vi "ReadVIInternal.vi"(1 "vi path":path) -> (0 "output cluster":T13)   [LabVIEW 2014]
uses:
  <vilib>/Utility/miscctls.llb/LVBoundsTypeDef.ctl
  <vilib>/Utility/miscctls.llb/LVPositionTypeDef.ctl
  <vilib>/Utility/miscctls.llb/LVRectTypeDef.ctl
  <vilib>/Utility/miscctls.llb/LVBreakpointStatusEnum.ctl
  <vilib>/Utility/miscctls.llb/LVDataSocketStatusTypeDef.ctl
  <vilib>/Utility/miscctls.llb/LVKeyNavTypeDef.ctl
  <vilib>/Utility/miscctls.llb/LVMinMaxIncTypeDef.ctl
  <vilib>/Utility/miscctls.llb/LVKeyTypeDef.ctl
  <vilib>/numeric/LVNumericRepresentation.ctl
  <vilib>/Utility/miscctls.llb/LVOutOfRangeActionTypeDef.ctl
  <vilib>/Utility/miscctls.llb/LVStringsAndValuesArrayTypeDef.ctl
  <vilib>/Utility/miscctls.llb/LVParallelSchedulesEnum.ctl
  <vilib>/Utility/traverseref.llb/VI Scripting - Traverse.lvlib
types:
  T1 = typedef "LVBoundsTypeDef.ctl" = cluster{"Width":u32, "Height":u32}
  T2 = typedef "LVPositionTypeDef.ctl" = cluster{"Left":i32, "Top":i32}
  T3 = typedef "LVRectTypeDef.ctl" = cluster{"Left":i16, "Top":i16, "Right":i16, "Bottom":i16}
  T4 = typedef "LVBreakpointStatusEnum.ctl" = enum8{"Cleared Break", "Enabled Break", "Disabled Break"}
  T5 = typedef "LVDataSocketStatusTypeDef.ctl" = cluster{"Code":enum32{"Invalid Status", "Unconnected", "Active", "Idle", "Error", "Connecting"}, "Text":string}
  T6 = typedef "LVKeyNavTypeDef.ctl" = cluster{"Control":bool, "Shift":bool, "Key":string}
  T7 = typedef "LVMinMaxIncTypeDef.ctl" = cluster{"Minimum":dbl, "Maximum":dbl, "Increment":dbl}
  T8 = typedef "LVKeyTypeDef.ctl" = cluster{"Focus":bool, "Control":bool, "Shift":bool, "Key":string}
  T9 = typedef "LVNumericRepresentation.ctl" = enum32{"Extended Precision", "Double Precision", "Single Precision", "Long", "Word", "Byte", "Unsigned Long", "Unsigned Word", "Unsigned Byte", "Complex Extended", "Complex Double", "Complex Single", "Quad", "Unsigned Quad", "Fixed-Point"}
  T10 = typedef "LVOutOfRangeActionTypeDef.ctl" = cluster{"Out of Range Action Minimum":u8, "Out of Range Action Maximum":u8, "Out of Range Action Increment":u8}
  T11 = typedef "LVStringsAndValuesArrayTypeDef.ctl" = cluster{"String":string, "Value":ext}[]
  T12 = typedef "LVParallelSchedulesEnum.ctl" = enum8{"Dynamic decreasing", "Dynamic fixed size", "Static block", "Static block-cyclic"}
  T13 = cluster{"Wire":cluster{"ClassID":u32, "ClassName":string, "IsOnBD?":bool, "Owner":cluster{bool, "UID":i32}, "OwningVI":refnum<vi>, "Bounds":T1, "Height":u32, "Width":u32, "Position":T2, "Left":i32, "Top":i32, "Selected":bool, "Bounds Rect":T3, "UID":i32, "BreakPtStatus":T4, "Desc":string, "Broken?":bool, "Joints[]":cluster{"Position":cluster{"h":i16, "v":i16}, "Flags":i32, "Type":enum32{"LooseEnd", "Endpoint", "Bend", "Junction"}, "Up Joint Index":i16, "Down Joint Index":i16, "Left Joint Index":i16, "Right Joint Index":i16}[], "Label":string, "Probe":refnum<vi>, "Terms[]":i32[], "Width":u32}[], cluster{"ClassID":u32, "ClassName":string, "IsOnBD?":bool, "Owner":cluster{bool, "UID":i32}, "OwningVI":refnum<vi>, "Bounds":T1, "Height":u32, "Width":u32, "Position":T2, "Left":i32, "Top":i32, "Selected":bool, "Bounds Rect":T3, "UID":i32, "Caption":string, "Coerce Dot?":bool, "Wire":i32, "Diagram":i32, "IsHidden":bool, "IsSource":bool, "Name":string}[], cluster{"ClassID":u32, "ClassName":string, "IsOnBD?":bool, "Owner":cluster{bool, "UID":i32}, "OwningVI":refnum<vi>, "Bounds":T1, "Height":u32, "Width":u32, "Position":T2, "Left":i32, "Top":i32, "Selected":bool, "Bounds Rect":T3, "UID":i32, "Input?":bool, "Name":string, "Term":i32}[], cluster{"ClassID":u32, "ClassName":string, "IsOnBD?":bool, "Owner":cluster{bool, "UID":i32}, "OwningVI":refnum<vi>, "Bounds":T1, "Height":u32, "Width":u32, "Position":T2, "Left":i32, "Top":i32, "Selected":bool, "Bounds Rect":T3, "UID":i32, "BreakPtStatus":T4, "Desc":string, "Label":string, "Style":string, "Terms[]":i32[], "FormExpr":string, "FormulaParameters[]":i32[]}[], cluster{"ClassID":u32, "ClassName":string, "IsOnBD?":bool, "Owner":cluster{bool, "UID":i32}, "OwningVI":refnum<vi>, "Bounds":T1, "Height":u32, "Width":u32, "Position":T2, "Left":i32, "Top":i32, "Selected":bool, "Bounds Rect":T3, "UID":i32, "BreakPtStatus":T4, "Desc":string, "Label":string, "Style":string, "Terms[]":i32[], "FormExpr":string, "FormulaParameters[]":i32[]}[], cluster{"ClassID":u32, "ClassName":string, "IsOnBD?":bool, "Owner":cluster{bool, "UID":i32}, "OwningVI":refnum<vi>, "Bounds":T1, "Height":u32, "Width":u32, "Position":T2, "Left":i32, "Top":i32, "Selected":bool, "Bounds Rect":T3, "UID":i32, "BreakPtStatus":T4, "Desc":string, "Label":string, "Style":string, "Terms[]":i32[], "TermHeight":i32, "Invert Inputs?[]":bool[], "Invert Output":bool, "Mode":u32}[], cluster{"ClassID":u32, "ClassName":string, "IsOnBD?":bool, "Owner":cluster{bool, "UID":i32}, "OwningVI":refnum<vi>, "Bounds":T1, "Height":u32, "Width":u32, "Position":T2, "Left":i32, "Top":i32, "Selected":bool, "Bounds Rect":T3, "UID":i32, "BreakPtStatus":T4, "Desc":string, "Label":string, "Style":string, "Terms[]":i32[], "TermHeight":i32, "InputCnt":i32, "InputTerms[]":i32[]}[], cluster{"ClassID":u32, "ClassName":string, "IsOnBD?":bool, "Owner":cluster{bool, "UID":i32}, "OwningVI":refnum<vi>, "Bounds":T1, "Height":u32, "Width":u32, "Position":T2, "Left":i32, "Top":i32, "Selected":bool, "Bounds Rect":T3, "UID":i32, "BreakPtStatus":T4, "Desc":string, "Label":string, "Style":string, "Terms[]":i32[], "TermHeight":i32, "OutputCnt":i32, "OutputTerms[]":i32[]}[], cluster{"ClassID":u32, "ClassName":string, "IsOnBD?":bool, "Owner":cluster{bool, "UID":i32}, "OwningVI":refnum<vi>, "Bounds":T1, "Height":u32, "Width":u32, "Position":T2, "Left":i32, "Top":i32, "Selected":bool, "Bounds Rect":T3, "UID":i32, "Auto-Update":bool, "Blinking":bool, "BuiltInMouseWheelSupport":enum16{"None", "On Hover", "On Key Focus", "On Hover or Key Focus"}, "Caption":refnum<vi>, "ControlIndex":i32, "CtrlRefNodes":refnum<vi>[], "FPB.BindingType":enum32{"Unbound", "Bound To PSP URL", "Bound To Variable Shortcut"}, "FPB.LEDVisible":bool, "FPB.Mode":enum32{"No PSP", "Read", "Write", "Write & Read"}, "FPB.URL":string, "FPB.Status":T5, "DtSktEnbld":bool, "DtSktTagVisible":bool, "DtSktMode":enum32{"No DataSocket", "Publish", "Subscribe", "Publish & Subscribe"}, "DtSktStatus":T5, "DtSktURL":string, "DefVal":variant, "Desc":string, "DisabledEnum":enum8{"Enabled", "Disabled", "Disabled and Grayed Out"}, "KeyNav":T6, "GrowInfo":cluster{"Can Grow Horiz":bool, "Can Grow Vert":bool, "Min Horiz":i16, "Min Vert":i16, "Max Horiz":i16, "Max Vert":i16}, "GrowInfoHorizOnly":bool, "GrowInfoVertOnly":bool, "GrowInfoMaxHoriz":i16, "GrowInfoMaxVert":i16, "GrowInfoMinHoriz":i16, "GrowInfoMinVert":i16, "HasCaption":bool, "Indicator":bool, "InvokeNodes":refnum<vi>[], "IsOnConPane":bool, "Typedef?":enum32{"not a typedef", "typedef", "strict typedef", "class private data"}, "Key Focus":bool, "Label":string, "Locals":refnum<vi>[], "OwningPane":refnum<vi>, "PropNodes":refnum<vi>[], "SkipTabbing":bool, "Style":u32, "SyncDisp":bool, "Terminal":i32, "TipStrip":string, "Typedef Path":path, "Typedef VI":refnum<vi>, "Value":variant, "Visible":bool, "Container Bounds":T1, "Height":u32, "Width":u32, "Is XControl?":bool, "Adapt To Source":bool, "Data Range":T7, "Increment":dbl, "Maximum":dbl, "Minimum":dbl, "DecKeyBind":T8, "IncKeyBind":T8, "Rep":T9, "OutOfRngAction":T10, "OutOfRngActInc":u8, "OutOfRngActMax":u8, "OutOfRngActMin":u8, "UnitLabel":refnum<vi>}[], cluster{"ClassID":u32, "ClassName":string, "IsOnBD?":bool, "Owner":cluster{bool, "UID":i32}, "OwningVI":refnum<vi>, "Bounds":T1, "Height":u32, "Width":u32, "Position":T2, "Left":i32, "Top":i32, "Selected":bool, "Bounds Rect":T3, "UID":i32, "Auto-Update":bool, "Blinking":bool, "BuiltInMouseWheelSupport":enum16{"None", "On Hover", "On Key Focus", "On Hover or Key Focus"}, "Caption":refnum<vi>, "ControlIndex":i32, "CtrlRefNodes":refnum<vi>[], "FPB.BindingType":enum32{"Unbound", "Bound To PSP URL", "Bound To Variable Shortcut"}, "FPB.LEDVisible":bool, "FPB.Mode":enum32{"No PSP", "Read", "Write", "Write & Read"}, "FPB.URL":string, "FPB.Status":T5, "DtSktEnbld":bool, "DtSktTagVisible":bool, "DtSktMode":enum32{"No DataSocket", "Publish", "Subscribe", "Publish & Subscribe"}, "DtSktStatus":T5, "DtSktURL":string, "DefVal":variant, "Desc":string, "DisabledEnum":enum8{"Enabled", "Disabled", "Disabled and Grayed Out"}, "KeyNav":T6, "GrowInfo":cluster{"Can Grow Horiz":bool, "Can Grow Vert":bool, "Min Horiz":i16, "Min Vert":i16, "Max Horiz":i16, "Max Vert":i16}, "GrowInfoHorizOnly":bool, "GrowInfoVertOnly":bool, "GrowInfoMaxHoriz":i16, "GrowInfoMaxVert":i16, "GrowInfoMinHoriz":i16, "GrowInfoMinVert":i16, "HasCaption":bool, "Indicator":bool, "InvokeNodes":refnum<vi>[], "IsOnConPane":bool, "Typedef?":enum32{"not a typedef", "typedef", "strict typedef", "class private data"}, "Key Focus":bool, "Label":string, "Locals":refnum<vi>[], "OwningPane":refnum<vi>, "PropNodes":refnum<vi>[], "SkipTabbing":bool, "Style":u32, "SyncDisp":bool, "Terminal":i32, "TipStrip":string, "Typedef Path":path, "Typedef VI":refnum<vi>, "Value":variant, "Visible":bool, "Container Bounds":T1, "Height":u32, "Width":u32, "Is XControl?":bool, "AllObjs[]":refnum<vi>[], "AutoSize":u32, "ClusterSize":T1, "ClustHeight":u32, "ClustWidth":u32, "Color":u32, "Controls[]":i32[], "Decos[]":refnum<vi>[]}[], cluster{"ClassID":u32, "ClassName":string, "IsOnBD?":bool, "Owner":cluster{bool, "UID":i32}, "OwningVI":refnum<vi>, "Bounds":T1, "Height":u32, "Width":u32, "Position":T2, "Left":i32, "Top":i32, "Selected":bool, "Bounds Rect":T3, "UID":i32, "Auto-Update":bool, "Blinking":bool, "BuiltInMouseWheelSupport":enum16{"None", "On Hover", "On Key Focus", "On Hover or Key Focus"}, "Caption":refnum<vi>, "ControlIndex":i32, "CtrlRefNodes":refnum<vi>[], "FPB.BindingType":enum32{"Unbound", "Bound To PSP URL", "Bound To Variable Shortcut"}, "FPB.LEDVisible":bool, "FPB.Mode":enum32{"No PSP", "Read", "Write", "Write & Read"}, "FPB.URL":string, "FPB.Status":T5, "DtSktEnbld":bool, "DtSktTagVisible":bool, "DtSktMode":enum32{"No DataSocket", "Publish", "Subscribe", "Publish & Subscribe"}, "DtSktStatus":T5, "DtSktURL":string, "DefVal":variant, "Desc":string, "DisabledEnum":enum8{"Enabled", "Disabled", "Disabled and Grayed Out"}, "KeyNav":T6, "GrowInfo":cluster{"Can Grow Horiz":bool, "Can Grow Vert":bool, "Min Horiz":i16, "Min Vert":i16, "Max Horiz":i16, "Max Vert":i16}, "GrowInfoHorizOnly":bool, "GrowInfoVertOnly":bool, "GrowInfoMaxHoriz":i16, "GrowInfoMaxVert":i16, "GrowInfoMinHoriz":i16, "GrowInfoMinVert":i16, "HasCaption":bool, "Indicator":bool, "InvokeNodes":refnum<vi>[], "IsOnConPane":bool, "Typedef?":enum32{"not a typedef", "typedef", "strict typedef", "class private data"}, "Key Focus":bool, "Label":string, "Locals":refnum<vi>[], "OwningPane":refnum<vi>, "PropNodes":refnum<vi>[], "SkipTabbing":bool, "Style":u32, "SyncDisp":bool, "Terminal":i32, "TipStrip":string, "Typedef Path":path, "Typedef VI":refnum<vi>, "Value":variant, "Visible":bool, "Container Bounds":T1, "Height":u32, "Width":u32, "Is XControl?":bool, "Array Element":refnum<vi>, "HorizScroll":bool, "Index Values":u32[], "Index Visible":bool, "Number of Columns":u32, "NumDims":u32, "Number of Rows":u32, "Selection Size []":u32[], "Selection Start []":u32[], "VertScroll":bool}[], cluster{"ClassID":u32, "ClassName":string, "IsOnBD?":bool, "Owner":cluster{bool, "UID":i32}, "OwningVI":refnum<vi>, "Bounds":T1, "Height":u32, "Width":u32, "Position":T2, "Left":i32, "Top":i32, "Selected":bool, "Bounds Rect":T3, "UID":i32, "Auto-Update":bool, "Desc":string, "Typedef?":enum32{"not a typedef", "typedef", "strict typedef", "class private data"}, "Label":string, "Terminal":i32, "TipStrip":string, "Typedef Path":path, "Typedef VI":refnum<vi>, "Value":variant, "Adapt To Entered Data":bool, "Representation":T9, "DigDisp":refnum<vi>, "Items[]":string[], "Allow Undefined Values?":bool, "Strings And Values[]":T11}[], cluster{"ClassID":u32, "ClassName":string, "IsOnBD?":bool, "Owner":cluster{bool, "UID":i32}, "OwningVI":refnum<vi>, "Bounds":T1, "Height":u32, "Width":u32, "Position":T2, "Left":i32, "Top":i32, "Selected":bool, "Bounds Rect":T3, "UID":i32, "BreakPtStatus":T4, "Desc":string, "Label":string, "Style":string, "Terms[]":i32[], "BadSubVILinkage":bool, "GrowTerms":string[], "SkipSbrtCall":bool, "CloseFPAfterCall":bool, "Open FP On Load":bool, "Show FP On Call":bool, "SuspendOnCall":bool, "TermVis":bool, "VIName":string, "VIPath":path, "VI Ref":refnum<vi>, "ViewAsIcon":bool}[], cluster{"ClassID":u32, "ClassName":string, "IsOnBD?":bool, "Owner":cluster{bool, "UID":i32}, "OwningVI":refnum<vi>, "Bounds":T1, "Height":u32, "Width":u32, "Position":T2, "Left":i32, "Top":i32, "Selected":bool, "Bounds Rect":T3, "UID":i32, "InsideTerms[]":i32[], "Outer Term":i32, "RightReg":i32}[], cluster{"ClassID":u32, "ClassName":string, "IsOnBD?":bool, "Owner":cluster{bool, "UID":i32}, "OwningVI":refnum<vi>, "Bounds":T1, "Height":u32, "Width":u32, "Position":T2, "Left":i32, "Top":i32, "Selected":bool, "Bounds Rect":T3, "UID":i32, "InsideTerms[]":i32[], "Outer Term":i32, "LeftRegs[]":i32[]}[], cluster{"ClassID":u32, "ClassName":string, "IsOnBD?":bool, "Owner":cluster{bool, "UID":i32}, "OwningVI":refnum<vi>, "Bounds":T1, "Height":u32, "Width":u32, "Position":T2, "Left":i32, "Top":i32, "Selected":bool, "Bounds Rect":T3, "UID":i32, "BreakPtStatus":T4, "Desc":string, "Label":string, "Style":string, "Terms[]":i32[], "AutoSize":bool, "Content Rect":T3, "Diagrams":refnum<vi>[], "Fix Contents":bool, "Frame Size":T1, "AutoSharedCloneAllocStrategyEnabled":bool, "PreAllocSharedClones":bool, "SubDiagLbl Vis":bool, "Tunnels[]":i32[], "Diagram":i32, "LpCounter":refnum<vi>, "ShiftRegs[]":i32[], "LpEndRef":refnum<vi>, "StopIfTrue":bool}[], cluster{"ClassID":u32, "ClassName":string, "IsOnBD?":bool, "Owner":cluster{bool, "UID":i32}, "OwningVI":refnum<vi>, "Bounds":T1, "Height":u32, "Width":u32, "Position":T2, "Left":i32, "Top":i32, "Selected":bool, "Bounds Rect":T3, "UID":i32, "BreakPtStatus":T4, "Desc":string, "Label":string, "Style":string, "Terms[]":i32[], "AutoSize":bool, "Content Rect":T3, "Diagrams":refnum<vi>[], "Fix Contents":bool, "Frame Size":T1, "AutoSharedCloneAllocStrategyEnabled":bool, "PreAllocSharedClones":bool, "SubDiagLbl Vis":bool, "Tunnels[]":i32[], "Diagram":i32, "LpCounter":refnum<vi>, "ShiftRegs[]":i32[], "ChunkSizeTunnel":refnum<vi>, "PTunnel":refnum<vi>, "HasConditionalTerm":bool, "DebuggingAllowed":bool, "IsParallelismEnabled":bool, "LpCount":refnum<vi>, "LpEndRef":refnum<vi>, "NumStaticParWorkers":i32, "ParallelSchedule":T12, "StopIfTrue":bool}[], cluster{"ClassID":u32, "ClassName":string, "IsOnBD?":bool, "Owner":cluster{bool, "UID":i32}, "OwningVI":refnum<vi>, "Bounds":T1, "Height":u32, "Width":u32, "Position":T2, "Left":i32, "Top":i32, "Selected":bool, "Bounds Rect":T3, "UID":i32, "AllObjs[]":refnum<vi>[], "BreakPtStatus":T4, "Color":u32, "Decos[]":refnum<vi>[], "FiringOrder":refnum<vi>[], "Nodes[]":refnum<vi>[], "SubDiag Label":refnum<vi>, "SubVIs[]":refnum<vi>[], "Wires[]":refnum<vi>[], "VisBounds":T1}[], cluster{"ClassID":u32, "ClassName":string, "IsOnBD?":bool, "Owner":cluster{bool, "UID":i32}, "OwningVI":refnum<vi>, "Bounds":T1, "Height":u32, "Width":u32, "Position":T2, "Left":i32, "Top":i32, "Selected":bool, "Bounds Rect":T3, "UID":i32, "AllObjs[]":refnum<vi>[], "Controls[]":i32[], "Decos[]":refnum<vi>[], "DeferPanUpdts":bool, "Panes[]":refnum<vi>[], "SelList[]":refnum<vi>[], "Splitters[]":refnum<vi>[]}[], cluster{"ClassID":u32, "ClassName":string, "IsOnBD?":bool, "Owner":cluster{bool, "UID":i32}, "OwningVI":refnum<vi>, "Bounds":T1, "Height":u32, "Width":u32, "Position":T2, "Left":i32, "Top":i32, "Selected":bool, "Bounds Rect":T3, "UID":i32, "InsideTerms[]":i32[], "Outer Term":i32}[]}
  T14 = cluster{"ClassID":u32, "ClassName":string, "IsOnBD?":bool, "Owner":cluster{bool, "UID":i32}, "OwningVI":refnum<vi>, "Bounds":T1, "Height":u32, "Width":u32, "Position":T2, "Left":i32, "Top":i32, "Selected":bool, "Bounds Rect":T3, "UID":i32, "BreakPtStatus":T4, "Desc":string, "Broken?":bool, "Joints[]":cluster{"Position":cluster{"h":i16, "v":i16}, "Flags":i32, "Type":enum32{"LooseEnd", "Endpoint", "Bend", "Junction"}, "Up Joint Index":i16, "Down Joint Index":i16, "Left Joint Index":i16, "Right Joint Index":i16}[], "Label":string, "Probe":refnum<vi>, "Terms[]":i32[], "Width":u32}
  T15 = cluster{"ClassID":u32, "ClassName":string, "IsOnBD?":bool, "Owner":cluster{bool, "UID":i32}, "OwningVI":refnum<vi>, "Bounds":T1, "Height":u32, "Width":u32, "Position":T2, "Left":i32, "Top":i32, "Selected":bool, "Bounds Rect":T3, "UID":i32, "Auto-Update":bool, "Blinking":bool, "BuiltInMouseWheelSupport":enum16{"None", "On Hover", "On Key Focus", "On Hover or Key Focus"}, "Caption":refnum<vi>, "ControlIndex":i32, "CtrlRefNodes":refnum<vi>[], "FPB.BindingType":enum32{"Unbound", "Bound To PSP URL", "Bound To Variable Shortcut"}, "FPB.LEDVisible":bool, "FPB.Mode":enum32{"No PSP", "Read", "Write", "Write & Read"}, "FPB.URL":string, "FPB.Status":T5, "DtSktEnbld":bool, "DtSktTagVisible":bool, "DtSktMode":enum32{"No DataSocket", "Publish", "Subscribe", "Publish & Subscribe"}, "DtSktStatus":T5, "DtSktURL":string, "DefVal":variant, "Desc":string, "DisabledEnum":enum8{"Enabled", "Disabled", "Disabled and Grayed Out"}, "KeyNav":T6, "GrowInfo":cluster{"Can Grow Horiz":bool, "Can Grow Vert":bool, "Min Horiz":i16, "Min Vert":i16, "Max Horiz":i16, "Max Vert":i16}, "GrowInfoHorizOnly":bool, "GrowInfoVertOnly":bool, "GrowInfoMaxHoriz":i16, "GrowInfoMaxVert":i16, "GrowInfoMinHoriz":i16, "GrowInfoMinVert":i16, "HasCaption":bool, "Indicator":bool, "InvokeNodes":refnum<vi>[], "IsOnConPane":bool, "Typedef?":enum32{"not a typedef", "typedef", "strict typedef", "class private data"}, "Key Focus":bool, "Label":string, "Locals":refnum<vi>[], "OwningPane":refnum<vi>, "PropNodes":refnum<vi>[], "SkipTabbing":bool, "Style":u32, "SyncDisp":bool, "Terminal":i32, "TipStrip":string, "Typedef Path":path, "Typedef VI":refnum<vi>, "Value":variant, "Visible":bool, "Container Bounds":T1, "Height":u32, "Width":u32, "Is XControl?":bool, "Array Element":refnum<vi>, "HorizScroll":bool, "Index Values":u32[], "Index Visible":bool, "Number of Columns":u32, "NumDims":u32, "Number of Rows":u32, "Selection Size []":u32[], "Selection Start []":u32[], "VertScroll":bool}
  T16 = cluster{"ClassID":u32, "ClassName":string, "IsOnBD?":bool, "Owner":cluster{bool, "UID":i32}, "OwningVI":refnum<vi>, "Bounds":T1, "Height":u32, "Width":u32, "Position":T2, "Left":i32, "Top":i32, "Selected":bool, "Bounds Rect":T3, "UID":i32, "BreakPtStatus":T4, "Desc":string, "Label":string, "Style":string, "Terms[]":i32[], "BadSubVILinkage":bool, "GrowTerms":string[], "SkipSbrtCall":bool, "CloseFPAfterCall":bool, "Open FP On Load":bool, "Show FP On Call":bool, "SuspendOnCall":bool, "TermVis":bool, "VIName":string, "VIPath":path, "VI Ref":refnum<vi>, "ViewAsIcon":bool}
  T17 = cluster{"ClassID":u32, "ClassName":string, "IsOnBD?":bool, "Owner":cluster{bool, "UID":i32}, "OwningVI":refnum<vi>, "Bounds":T1, "Height":u32, "Width":u32, "Position":T2, "Left":i32, "Top":i32, "Selected":bool, "Bounds Rect":T3, "UID":i32, "AllObjs[]":refnum<vi>[], "Controls[]":i32[], "Decos[]":refnum<vi>[], "DeferPanUpdts":bool, "Panes[]":refnum<vi>[], "SelList[]":refnum<vi>[], "Splitters[]":refnum<vi>[]}
  T18 = cluster{"ClassID":u32, "ClassName":string, "IsOnBD?":bool, "Owner":cluster{bool, "UID":i32}, "OwningVI":refnum<vi>, "Bounds":T1, "Height":u32, "Width":u32, "Position":T2, "Left":i32, "Top":i32, "Selected":bool, "Bounds Rect":T3, "UID":i32, "Caption":string, "Coerce Dot?":bool, "Wire":i32, "Diagram":i32, "IsHidden":bool, "IsSource":bool, "Name":string}
  T19 = cluster{"ClassID":u32, "ClassName":string, "IsOnBD?":bool, "Owner":cluster{bool, "UID":i32}, "OwningVI":refnum<vi>, "Bounds":T1, "Height":u32, "Width":u32, "Position":T2, "Left":i32, "Top":i32, "Selected":bool, "Bounds Rect":T3, "UID":i32, "Input?":bool, "Name":string, "Term":i32}
  T20 = cluster{"ClassID":u32, "ClassName":string, "IsOnBD?":bool, "Owner":cluster{bool, "UID":i32}, "OwningVI":refnum<vi>, "Bounds":T1, "Height":u32, "Width":u32, "Position":T2, "Left":i32, "Top":i32, "Selected":bool, "Bounds Rect":T3, "UID":i32, "BreakPtStatus":T4, "Desc":string, "Label":string, "Style":string, "Terms[]":i32[], "FormExpr":string, "FormulaParameters[]":i32[]}
  T21 = cluster{"ClassID":u32, "ClassName":string, "IsOnBD?":bool, "Owner":cluster{bool, "UID":i32}, "OwningVI":refnum<vi>, "Bounds":T1, "Height":u32, "Width":u32, "Position":T2, "Left":i32, "Top":i32, "Selected":bool, "Bounds Rect":T3, "UID":i32, "BreakPtStatus":T4, "Desc":string, "Label":string, "Style":string, "Terms[]":i32[], "TermHeight":i32, "Invert Inputs?[]":bool[], "Invert Output":bool, "Mode":u32}
  T22 = cluster{"ClassID":u32, "ClassName":string, "IsOnBD?":bool, "Owner":cluster{bool, "UID":i32}, "OwningVI":refnum<vi>, "Bounds":T1, "Height":u32, "Width":u32, "Position":T2, "Left":i32, "Top":i32, "Selected":bool, "Bounds Rect":T3, "UID":i32, "BreakPtStatus":T4, "Desc":string, "Label":string, "Style":string, "Terms[]":i32[], "TermHeight":i32, "InputCnt":i32, "InputTerms[]":i32[]}
  T23 = cluster{"ClassID":u32, "ClassName":string, "IsOnBD?":bool, "Owner":cluster{bool, "UID":i32}, "OwningVI":refnum<vi>, "Bounds":T1, "Height":u32, "Width":u32, "Position":T2, "Left":i32, "Top":i32, "Selected":bool, "Bounds Rect":T3, "UID":i32, "BreakPtStatus":T4, "Desc":string, "Label":string, "Style":string, "Terms[]":i32[], "TermHeight":i32, "OutputCnt":i32, "OutputTerms[]":i32[]}
  T24 = cluster{"ClassID":u32, "ClassName":string, "IsOnBD?":bool, "Owner":cluster{bool, "UID":i32}, "OwningVI":refnum<vi>, "Bounds":T1, "Height":u32, "Width":u32, "Position":T2, "Left":i32, "Top":i32, "Selected":bool, "Bounds Rect":T3, "UID":i32, "Auto-Update":bool, "Blinking":bool, "BuiltInMouseWheelSupport":enum16{"None", "On Hover", "On Key Focus", "On Hover or Key Focus"}, "Caption":refnum<vi>, "ControlIndex":i32, "CtrlRefNodes":refnum<vi>[], "FPB.BindingType":enum32{"Unbound", "Bound To PSP URL", "Bound To Variable Shortcut"}, "FPB.LEDVisible":bool, "FPB.Mode":enum32{"No PSP", "Read", "Write", "Write & Read"}, "FPB.URL":string, "FPB.Status":T5, "DtSktEnbld":bool, "DtSktTagVisible":bool, "DtSktMode":enum32{"No DataSocket", "Publish", "Subscribe", "Publish & Subscribe"}, "DtSktStatus":T5, "DtSktURL":string, "DefVal":variant, "Desc":string, "DisabledEnum":enum8{"Enabled", "Disabled", "Disabled and Grayed Out"}, "KeyNav":T6, "GrowInfo":cluster{"Can Grow Horiz":bool, "Can Grow Vert":bool, "Min Horiz":i16, "Min Vert":i16, "Max Horiz":i16, "Max Vert":i16}, "GrowInfoHorizOnly":bool, "GrowInfoVertOnly":bool, "GrowInfoMaxHoriz":i16, "GrowInfoMaxVert":i16, "GrowInfoMinHoriz":i16, "GrowInfoMinVert":i16, "HasCaption":bool, "Indicator":bool, "InvokeNodes":refnum<vi>[], "IsOnConPane":bool, "Typedef?":enum32{"not a typedef", "typedef", "strict typedef", "class private data"}, "Key Focus":bool, "Label":string, "Locals":refnum<vi>[], "OwningPane":refnum<vi>, "PropNodes":refnum<vi>[], "SkipTabbing":bool, "Style":u32, "SyncDisp":bool, "Terminal":i32, "TipStrip":string, "Typedef Path":path, "Typedef VI":refnum<vi>, "Value":variant, "Visible":bool, "Container Bounds":T1, "Height":u32, "Width":u32, "Is XControl?":bool, "Adapt To Source":bool, "Data Range":T7, "Increment":dbl, "Maximum":dbl, "Minimum":dbl, "DecKeyBind":T8, "IncKeyBind":T8, "Rep":T9, "OutOfRngAction":T10, "OutOfRngActInc":u8, "OutOfRngActMax":u8, "OutOfRngActMin":u8, "UnitLabel":refnum<vi>}
  T25 = cluster{"ClassID":u32, "ClassName":string, "IsOnBD?":bool, "Owner":cluster{bool, "UID":i32}, "OwningVI":refnum<vi>, "Bounds":T1, "Height":u32, "Width":u32, "Position":T2, "Left":i32, "Top":i32, "Selected":bool, "Bounds Rect":T3, "UID":i32, "Auto-Update":bool, "Blinking":bool, "BuiltInMouseWheelSupport":enum16{"None", "On Hover", "On Key Focus", "On Hover or Key Focus"}, "Caption":refnum<vi>, "ControlIndex":i32, "CtrlRefNodes":refnum<vi>[], "FPB.BindingType":enum32{"Unbound", "Bound To PSP URL", "Bound To Variable Shortcut"}, "FPB.LEDVisible":bool, "FPB.Mode":enum32{"No PSP", "Read", "Write", "Write & Read"}, "FPB.URL":string, "FPB.Status":T5, "DtSktEnbld":bool, "DtSktTagVisible":bool, "DtSktMode":enum32{"No DataSocket", "Publish", "Subscribe", "Publish & Subscribe"}, "DtSktStatus":T5, "DtSktURL":string, "DefVal":variant, "Desc":string, "DisabledEnum":enum8{"Enabled", "Disabled", "Disabled and Grayed Out"}, "KeyNav":T6, "GrowInfo":cluster{"Can Grow Horiz":bool, "Can Grow Vert":bool, "Min Horiz":i16, "Min Vert":i16, "Max Horiz":i16, "Max Vert":i16}, "GrowInfoHorizOnly":bool, "GrowInfoVertOnly":bool, "GrowInfoMaxHoriz":i16, "GrowInfoMaxVert":i16, "GrowInfoMinHoriz":i16, "GrowInfoMinVert":i16, "HasCaption":bool, "Indicator":bool, "InvokeNodes":refnum<vi>[], "IsOnConPane":bool, "Typedef?":enum32{"not a typedef", "typedef", "strict typedef", "class private data"}, "Key Focus":bool, "Label":string, "Locals":refnum<vi>[], "OwningPane":refnum<vi>, "PropNodes":refnum<vi>[], "SkipTabbing":bool, "Style":u32, "SyncDisp":bool, "Terminal":i32, "TipStrip":string, "Typedef Path":path, "Typedef VI":refnum<vi>, "Value":variant, "Visible":bool, "Container Bounds":T1, "Height":u32, "Width":u32, "Is XControl?":bool, "AllObjs[]":refnum<vi>[], "AutoSize":u32, "ClusterSize":T1, "ClustHeight":u32, "ClustWidth":u32, "Color":u32, "Controls[]":i32[], "Decos[]":refnum<vi>[]}
  T26 = cluster{"ClassID":u32, "ClassName":string, "IsOnBD?":bool, "Owner":cluster{bool, "UID":i32}, "OwningVI":refnum<vi>, "Bounds":T1, "Height":u32, "Width":u32, "Position":T2, "Left":i32, "Top":i32, "Selected":bool, "Bounds Rect":T3, "UID":i32, "Auto-Update":bool, "Desc":string, "Typedef?":enum32{"not a typedef", "typedef", "strict typedef", "class private data"}, "Label":string, "Terminal":i32, "TipStrip":string, "Typedef Path":path, "Typedef VI":refnum<vi>, "Value":variant, "Adapt To Entered Data":bool, "Representation":T9, "DigDisp":refnum<vi>, "Items[]":string[], "Allow Undefined Values?":bool, "Strings And Values[]":T11}
  T27 = cluster{"ClassID":u32, "ClassName":string, "IsOnBD?":bool, "Owner":cluster{bool, "UID":i32}, "OwningVI":refnum<vi>, "Bounds":T1, "Height":u32, "Width":u32, "Position":T2, "Left":i32, "Top":i32, "Selected":bool, "Bounds Rect":T3, "UID":i32, "InsideTerms[]":i32[], "Outer Term":i32, "RightReg":i32}
  T28 = cluster{"ClassID":u32, "ClassName":string, "IsOnBD?":bool, "Owner":cluster{bool, "UID":i32}, "OwningVI":refnum<vi>, "Bounds":T1, "Height":u32, "Width":u32, "Position":T2, "Left":i32, "Top":i32, "Selected":bool, "Bounds Rect":T3, "UID":i32, "InsideTerms[]":i32[], "Outer Term":i32, "LeftRegs[]":i32[]}
  T29 = cluster{"ClassID":u32, "ClassName":string, "IsOnBD?":bool, "Owner":cluster{bool, "UID":i32}, "OwningVI":refnum<vi>, "Bounds":T1, "Height":u32, "Width":u32, "Position":T2, "Left":i32, "Top":i32, "Selected":bool, "Bounds Rect":T3, "UID":i32, "BreakPtStatus":T4, "Desc":string, "Label":string, "Style":string, "Terms[]":i32[], "AutoSize":bool, "Content Rect":T3, "Diagrams":refnum<vi>[], "Fix Contents":bool, "Frame Size":T1, "AutoSharedCloneAllocStrategyEnabled":bool, "PreAllocSharedClones":bool, "SubDiagLbl Vis":bool, "Tunnels[]":i32[], "Diagram":i32, "LpCounter":refnum<vi>, "ShiftRegs[]":i32[], "LpEndRef":refnum<vi>, "StopIfTrue":bool}
  T30 = cluster{"ClassID":u32, "ClassName":string, "IsOnBD?":bool, "Owner":cluster{bool, "UID":i32}, "OwningVI":refnum<vi>, "Bounds":T1, "Height":u32, "Width":u32, "Position":T2, "Left":i32, "Top":i32, "Selected":bool, "Bounds Rect":T3, "UID":i32, "BreakPtStatus":T4, "Desc":string, "Label":string, "Style":string, "Terms[]":i32[], "AutoSize":bool, "Content Rect":T3, "Diagrams":refnum<vi>[], "Fix Contents":bool, "Frame Size":T1, "AutoSharedCloneAllocStrategyEnabled":bool, "PreAllocSharedClones":bool, "SubDiagLbl Vis":bool, "Tunnels[]":i32[], "Diagram":i32, "LpCounter":refnum<vi>, "ShiftRegs[]":i32[], "ChunkSizeTunnel":refnum<vi>, "PTunnel":refnum<vi>, "HasConditionalTerm":bool, "DebuggingAllowed":bool, "IsParallelismEnabled":bool, "LpCount":refnum<vi>, "LpEndRef":refnum<vi>, "NumStaticParWorkers":i32, "ParallelSchedule":T12, "StopIfTrue":bool}
  T31 = cluster{"ClassID":u32, "ClassName":string, "IsOnBD?":bool, "Owner":cluster{bool, "UID":i32}, "OwningVI":refnum<vi>, "Bounds":T1, "Height":u32, "Width":u32, "Position":T2, "Left":i32, "Top":i32, "Selected":bool, "Bounds Rect":T3, "UID":i32, "AllObjs[]":refnum<vi>[], "BreakPtStatus":T4, "Color":u32, "Decos[]":refnum<vi>[], "FiringOrder":refnum<vi>[], "Nodes[]":refnum<vi>[], "SubDiag Label":refnum<vi>, "SubVIs[]":refnum<vi>[], "Wires[]":refnum<vi>[], "VisBounds":T1}
  T32 = cluster{"ClassID":u32, "ClassName":string, "IsOnBD?":bool, "Owner":cluster{bool, "UID":i32}, "OwningVI":refnum<vi>, "Bounds":T1, "Height":u32, "Width":u32, "Position":T2, "Left":i32, "Top":i32, "Selected":bool, "Bounds Rect":T3, "UID":i32, "InsideTerms[]":i32[], "Outer Term":i32}
  T33 = cluster{cluster{"ClassID":u32, "ClassName":string, "IsOnBD?":bool, "Owner":cluster{bool, "UID":i32}, "OwningVI":refnum<vi>, "Bounds":T1, "Height":u32, "Width":u32, "Position":T2, "Left":i32, "Top":i32, "Selected":bool, "Bounds Rect":T3, "UID":i32, "BreakPtStatus":T4, "Desc":string, "Broken?":bool, "Joints[]":cluster{"Position":cluster{"h":i16, "v":i16}, "Flags":i32, "Type":enum32{"LooseEnd", "Endpoint", "Bend", "Junction"}, "Up Joint Index":i16, "Down Joint Index":i16, "Left Joint Index":i16, "Right Joint Index":i16}[], "Label":string, "Probe":refnum<vi>, "Terms[]":i32[], "Width":u32}[], cluster{"ClassID":u32, "ClassName":string, "IsOnBD?":bool, "Owner":cluster{bool, "UID":i32}, "OwningVI":refnum<vi>, "Bounds":T1, "Height":u32, "Width":u32, "Position":T2, "Left":i32, "Top":i32, "Selected":bool, "Bounds Rect":T3, "UID":i32, "Caption":string, "Coerce Dot?":bool, "Wire":i32, "Diagram":i32, "IsHidden":bool, "IsSource":bool, "Name":string}[], cluster{"ClassID":u32, "ClassName":string, "IsOnBD?":bool, "Owner":cluster{bool, "UID":i32}, "OwningVI":refnum<vi>, "Bounds":T1, "Height":u32, "Width":u32, "Position":T2, "Left":i32, "Top":i32, "Selected":bool, "Bounds Rect":T3, "UID":i32, "Input?":bool, "Name":string, "Term":i32}[], cluster{"ClassID":u32, "ClassName":string, "IsOnBD?":bool, "Owner":cluster{bool, "UID":i32}, "OwningVI":refnum<vi>, "Bounds":T1, "Height":u32, "Width":u32, "Position":T2, "Left":i32, "Top":i32, "Selected":bool, "Bounds Rect":T3, "UID":i32, "BreakPtStatus":T4, "Desc":string, "Label":string, "Style":string, "Terms[]":i32[], "FormExpr":string, "FormulaParameters[]":i32[]}[], cluster{"ClassID":u32, "ClassName":string, "IsOnBD?":bool, "Owner":cluster{bool, "UID":i32}, "OwningVI":refnum<vi>, "Bounds":T1, "Height":u32, "Width":u32, "Position":T2, "Left":i32, "Top":i32, "Selected":bool, "Bounds Rect":T3, "UID":i32, "BreakPtStatus":T4, "Desc":string, "Label":string, "Style":string, "Terms[]":i32[], "FormExpr":string, "FormulaParameters[]":i32[]}[], cluster{"ClassID":u32, "ClassName":string, "IsOnBD?":bool, "Owner":cluster{bool, "UID":i32}, "OwningVI":refnum<vi>, "Bounds":T1, "Height":u32, "Width":u32, "Position":T2, "Left":i32, "Top":i32, "Selected":bool, "Bounds Rect":T3, "UID":i32, "BreakPtStatus":T4, "Desc":string, "Label":string, "Style":string, "Terms[]":i32[], "TermHeight":i32, "Invert Inputs?[]":bool[], "Invert Output":bool, "Mode":u32}[], cluster{"ClassID":u32, "ClassName":string, "IsOnBD?":bool, "Owner":cluster{bool, "UID":i32}, "OwningVI":refnum<vi>, "Bounds":T1, "Height":u32, "Width":u32, "Position":T2, "Left":i32, "Top":i32, "Selected":bool, "Bounds Rect":T3, "UID":i32, "BreakPtStatus":T4, "Desc":string, "Label":string, "Style":string, "Terms[]":i32[], "TermHeight":i32, "InputCnt":i32, "InputTerms[]":i32[]}[], cluster{"ClassID":u32, "ClassName":string, "IsOnBD?":bool, "Owner":cluster{bool, "UID":i32}, "OwningVI":refnum<vi>, "Bounds":T1, "Height":u32, "Width":u32, "Position":T2, "Left":i32, "Top":i32, "Selected":bool, "Bounds Rect":T3, "UID":i32, "BreakPtStatus":T4, "Desc":string, "Label":string, "Style":string, "Terms[]":i32[], "TermHeight":i32, "OutputCnt":i32, "OutputTerms[]":i32[]}[], cluster{"ClassID":u32, "ClassName":string, "IsOnBD?":bool, "Owner":cluster{bool, "UID":i32}, "OwningVI":refnum<vi>, "Bounds":T1, "Height":u32, "Width":u32, "Position":T2, "Left":i32, "Top":i32, "Selected":bool, "Bounds Rect":T3, "UID":i32, "Auto-Update":bool, "Blinking":bool, "BuiltInMouseWheelSupport":enum16{"None", "On Hover", "On Key Focus", "On Hover or Key Focus"}, "Caption":refnum<vi>, "ControlIndex":i32, "CtrlRefNodes":refnum<vi>[], "FPB.BindingType":enum32{"Unbound", "Bound To PSP URL", "Bound To Variable Shortcut"}, "FPB.LEDVisible":bool, "FPB.Mode":enum32{"No PSP", "Read", "Write", "Write & Read"}, "FPB.URL":string, "FPB.Status":T5, "DtSktEnbld":bool, "DtSktTagVisible":bool, "DtSktMode":enum32{"No DataSocket", "Publish", "Subscribe", "Publish & Subscribe"}, "DtSktStatus":T5, "DtSktURL":string, "DefVal":variant, "Desc":string, "DisabledEnum":enum8{"Enabled", "Disabled", "Disabled and Grayed Out"}, "KeyNav":T6, "GrowInfo":cluster{"Can Grow Horiz":bool, "Can Grow Vert":bool, "Min Horiz":i16, "Min Vert":i16, "Max Horiz":i16, "Max Vert":i16}, "GrowInfoHorizOnly":bool, "GrowInfoVertOnly":bool, "GrowInfoMaxHoriz":i16, "GrowInfoMaxVert":i16, "GrowInfoMinHoriz":i16, "GrowInfoMinVert":i16, "HasCaption":bool, "Indicator":bool, "InvokeNodes":refnum<vi>[], "IsOnConPane":bool, "Typedef?":enum32{"not a typedef", "typedef", "strict typedef", "class private data"}, "Key Focus":bool, "Label":string, "Locals":refnum<vi>[], "OwningPane":refnum<vi>, "PropNodes":refnum<vi>[], "SkipTabbing":bool, "Style":u32, "SyncDisp":bool, "Terminal":i32, "TipStrip":string, "Typedef Path":path, "Typedef VI":refnum<vi>, "Value":variant, "Visible":bool, "Container Bounds":T1, "Height":u32, "Width":u32, "Is XControl?":bool, "Adapt To Source":bool, "Data Range":T7, "Increment":dbl, "Maximum":dbl, "Minimum":dbl, "DecKeyBind":T8, "IncKeyBind":T8, "Rep":T9, "OutOfRngAction":T10, "OutOfRngActInc":u8, "OutOfRngActMax":u8, "OutOfRngActMin":u8, "UnitLabel":refnum<vi>}[], cluster{"ClassID":u32, "ClassName":string, "IsOnBD?":bool, "Owner":cluster{bool, "UID":i32}, "OwningVI":refnum<vi>, "Bounds":T1, "Height":u32, "Width":u32, "Position":T2, "Left":i32, "Top":i32, "Selected":bool, "Bounds Rect":T3, "UID":i32, "Auto-Update":bool, "Blinking":bool, "BuiltInMouseWheelSupport":enum16{"None", "On Hover", "On Key Focus", "On Hover or Key Focus"}, "Caption":refnum<vi>, "ControlIndex":i32, "CtrlRefNodes":refnum<vi>[], "FPB.BindingType":enum32{"Unbound", "Bound To PSP URL", "Bound To Variable Shortcut"}, "FPB.LEDVisible":bool, "FPB.Mode":enum32{"No PSP", "Read", "Write", "Write & Read"}, "FPB.URL":string, "FPB.Status":T5, "DtSktEnbld":bool, "DtSktTagVisible":bool, "DtSktMode":enum32{"No DataSocket", "Publish", "Subscribe", "Publish & Subscribe"}, "DtSktStatus":T5, "DtSktURL":string, "DefVal":variant, "Desc":string, "DisabledEnum":enum8{"Enabled", "Disabled", "Disabled and Grayed Out"}, "KeyNav":T6, "GrowInfo":cluster{"Can Grow Horiz":bool, "Can Grow Vert":bool, "Min Horiz":i16, "Min Vert":i16, "Max Horiz":i16, "Max Vert":i16}, "GrowInfoHorizOnly":bool, "GrowInfoVertOnly":bool, "GrowInfoMaxHoriz":i16, "GrowInfoMaxVert":i16, "GrowInfoMinHoriz":i16, "GrowInfoMinVert":i16, "HasCaption":bool, "Indicator":bool, "InvokeNodes":refnum<vi>[], "IsOnConPane":bool, "Typedef?":enum32{"not a typedef", "typedef", "strict typedef", "class private data"}, "Key Focus":bool, "Label":string, "Locals":refnum<vi>[], "OwningPane":refnum<vi>, "PropNodes":refnum<vi>[], "SkipTabbing":bool, "Style":u32, "SyncDisp":bool, "Terminal":i32, "TipStrip":string, "Typedef Path":path, "Typedef VI":refnum<vi>, "Value":variant, "Visible":bool, "Container Bounds":T1, "Height":u32, "Width":u32, "Is XControl?":bool, "AllObjs[]":refnum<vi>[], "AutoSize":u32, "ClusterSize":T1, "ClustHeight":u32, "ClustWidth":u32, "Color":u32, "Controls[]":i32[], "Decos[]":refnum<vi>[]}[], cluster{"ClassID":u32, "ClassName":string, "IsOnBD?":bool, "Owner":cluster{bool, "UID":i32}, "OwningVI":refnum<vi>, "Bounds":T1, "Height":u32, "Width":u32, "Position":T2, "Left":i32, "Top":i32, "Selected":bool, "Bounds Rect":T3, "UID":i32, "Auto-Update":bool, "Blinking":bool, "BuiltInMouseWheelSupport":enum16{"None", "On Hover", "On Key Focus", "On Hover or Key Focus"}, "Caption":refnum<vi>, "ControlIndex":i32, "CtrlRefNodes":refnum<vi>[], "FPB.BindingType":enum32{"Unbound", "Bound To PSP URL", "Bound To Variable Shortcut"}, "FPB.LEDVisible":bool, "FPB.Mode":enum32{"No PSP", "Read", "Write", "Write & Read"}, "FPB.URL":string, "FPB.Status":T5, "DtSktEnbld":bool, "DtSktTagVisible":bool, "DtSktMode":enum32{"No DataSocket", "Publish", "Subscribe", "Publish & Subscribe"}, "DtSktStatus":T5, "DtSktURL":string, "DefVal":variant, "Desc":string, "DisabledEnum":enum8{"Enabled", "Disabled", "Disabled and Grayed Out"}, "KeyNav":T6, "GrowInfo":cluster{"Can Grow Horiz":bool, "Can Grow Vert":bool, "Min Horiz":i16, "Min Vert":i16, "Max Horiz":i16, "Max Vert":i16}, "GrowInfoHorizOnly":bool, "GrowInfoVertOnly":bool, "GrowInfoMaxHoriz":i16, "GrowInfoMaxVert":i16, "GrowInfoMinHoriz":i16, "GrowInfoMinVert":i16, "HasCaption":bool, "Indicator":bool, "InvokeNodes":refnum<vi>[], "IsOnConPane":bool, "Typedef?":enum32{"not a typedef", "typedef", "strict typedef", "class private data"}, "Key Focus":bool, "Label":string, "Locals":refnum<vi>[], "OwningPane":refnum<vi>, "PropNodes":refnum<vi>[], "SkipTabbing":bool, "Style":u32, "SyncDisp":bool, "Terminal":i32, "TipStrip":string, "Typedef Path":path, "Typedef VI":refnum<vi>, "Value":variant, "Visible":bool, "Container Bounds":T1, "Height":u32, "Width":u32, "Is XControl?":bool, "Array Element":refnum<vi>, "HorizScroll":bool, "Index Values":u32[], "Index Visible":bool, "Number of Columns":u32, "NumDims":u32, "Number of Rows":u32, "Selection Size []":u32[], "Selection Start []":u32[], "VertScroll":bool}[], cluster{"ClassID":u32, "ClassName":string, "IsOnBD?":bool, "Owner":cluster{bool, "UID":i32}, "OwningVI":refnum<vi>, "Bounds":T1, "Height":u32, "Width":u32, "Position":T2, "Left":i32, "Top":i32, "Selected":bool, "Bounds Rect":T3, "UID":i32, "Auto-Update":bool, "Desc":string, "Typedef?":enum32{"not a typedef", "typedef", "strict typedef", "class private data"}, "Label":string, "Terminal":i32, "TipStrip":string, "Typedef Path":path, "Typedef VI":refnum<vi>, "Value":variant, "Adapt To Entered Data":bool, "Representation":T9, "DigDisp":refnum<vi>, "Items[]":string[], "Allow Undefined Values?":bool, "Strings And Values[]":T11}[], cluster{"ClassID":u32, "ClassName":string, "IsOnBD?":bool, "Owner":cluster{bool, "UID":i32}, "OwningVI":refnum<vi>, "Bounds":T1, "Height":u32, "Width":u32, "Position":T2, "Left":i32, "Top":i32, "Selected":bool, "Bounds Rect":T3, "UID":i32, "BreakPtStatus":T4, "Desc":string, "Label":string, "Style":string, "Terms[]":i32[], "BadSubVILinkage":bool, "GrowTerms":string[], "SkipSbrtCall":bool, "CloseFPAfterCall":bool, "Open FP On Load":bool, "Show FP On Call":bool, "SuspendOnCall":bool, "TermVis":bool, "VIName":string, "VIPath":path, "VI Ref":refnum<vi>, "ViewAsIcon":bool}[], cluster{"ClassID":u32, "ClassName":string, "IsOnBD?":bool, "Owner":cluster{bool, "UID":i32}, "OwningVI":refnum<vi>, "Bounds":T1, "Height":u32, "Width":u32, "Position":T2, "Left":i32, "Top":i32, "Selected":bool, "Bounds Rect":T3, "UID":i32, "InsideTerms[]":i32[], "Outer Term":i32, "RightReg":i32}[], cluster{"ClassID":u32, "ClassName":string, "IsOnBD?":bool, "Owner":cluster{bool, "UID":i32}, "OwningVI":refnum<vi>, "Bounds":T1, "Height":u32, "Width":u32, "Position":T2, "Left":i32, "Top":i32, "Selected":bool, "Bounds Rect":T3, "UID":i32, "InsideTerms[]":i32[], "Outer Term":i32, "LeftRegs[]":i32[]}[], cluster{"ClassID":u32, "ClassName":string, "IsOnBD?":bool, "Owner":cluster{bool, "UID":i32}, "OwningVI":refnum<vi>, "Bounds":T1, "Height":u32, "Width":u32, "Position":T2, "Left":i32, "Top":i32, "Selected":bool, "Bounds Rect":T3, "UID":i32, "BreakPtStatus":T4, "Desc":string, "Label":string, "Style":string, "Terms[]":i32[], "AutoSize":bool, "Content Rect":T3, "Diagrams":refnum<vi>[], "Fix Contents":bool, "Frame Size":T1, "AutoSharedCloneAllocStrategyEnabled":bool, "PreAllocSharedClones":bool, "SubDiagLbl Vis":bool, "Tunnels[]":i32[], "Diagram":i32, "LpCounter":refnum<vi>, "ShiftRegs[]":i32[], "LpEndRef":refnum<vi>, "StopIfTrue":bool}[], cluster{"ClassID":u32, "ClassName":string, "IsOnBD?":bool, "Owner":cluster{bool, "UID":i32}, "OwningVI":refnum<vi>, "Bounds":T1, "Height":u32, "Width":u32, "Position":T2, "Left":i32, "Top":i32, "Selected":bool, "Bounds Rect":T3, "UID":i32, "BreakPtStatus":T4, "Desc":string, "Label":string, "Style":string, "Terms[]":i32[], "AutoSize":bool, "Content Rect":T3, "Diagrams":refnum<vi>[], "Fix Contents":bool, "Frame Size":T1, "AutoSharedCloneAllocStrategyEnabled":bool, "PreAllocSharedClones":bool, "SubDiagLbl Vis":bool, "Tunnels[]":i32[], "Diagram":i32, "LpCounter":refnum<vi>, "ShiftRegs[]":i32[], "ChunkSizeTunnel":refnum<vi>, "PTunnel":refnum<vi>, "HasConditionalTerm":bool, "DebuggingAllowed":bool, "IsParallelismEnabled":bool, "LpCount":refnum<vi>, "LpEndRef":refnum<vi>, "NumStaticParWorkers":i32, "ParallelSchedule":T12, "StopIfTrue":bool}[], cluster{"ClassID":u32, "ClassName":string, "IsOnBD?":bool, "Owner":cluster{bool, "UID":i32}, "OwningVI":refnum<vi>, "Bounds":T1, "Height":u32, "Width":u32, "Position":T2, "Left":i32, "Top":i32, "Selected":bool, "Bounds Rect":T3, "UID":i32, "AllObjs[]":refnum<vi>[], "BreakPtStatus":T4, "Color":u32, "Decos[]":refnum<vi>[], "FiringOrder":refnum<vi>[], "Nodes[]":refnum<vi>[], "SubDiag Label":refnum<vi>, "SubVIs[]":refnum<vi>[], "Wires[]":refnum<vi>[], "VisBounds":T1}[], cluster{"ClassID":u32, "ClassName":string, "IsOnBD?":bool, "Owner":cluster{bool, "UID":i32}, "OwningVI":refnum<vi>, "Bounds":T1, "Height":u32, "Width":u32, "Position":T2, "Left":i32, "Top":i32, "Selected":bool, "Bounds Rect":T3, "UID":i32, "AllObjs[]":refnum<vi>[], "Controls[]":i32[], "Decos[]":refnum<vi>[], "DeferPanUpdts":bool, "Panes[]":refnum<vi>[], "SelList[]":refnum<vi>[], "Splitters[]":refnum<vi>[]}[], cluster{"ClassID":u32, "ClassName":string, "IsOnBD?":bool, "Owner":cluster{bool, "UID":i32}, "OwningVI":refnum<vi>, "Bounds":T1, "Height":u32, "Width":u32, "Position":T2, "Left":i32, "Top":i32, "Selected":bool, "Bounds Rect":T3, "UID":i32, "InsideTerms[]":i32[], "Outer Term":i32}[]}
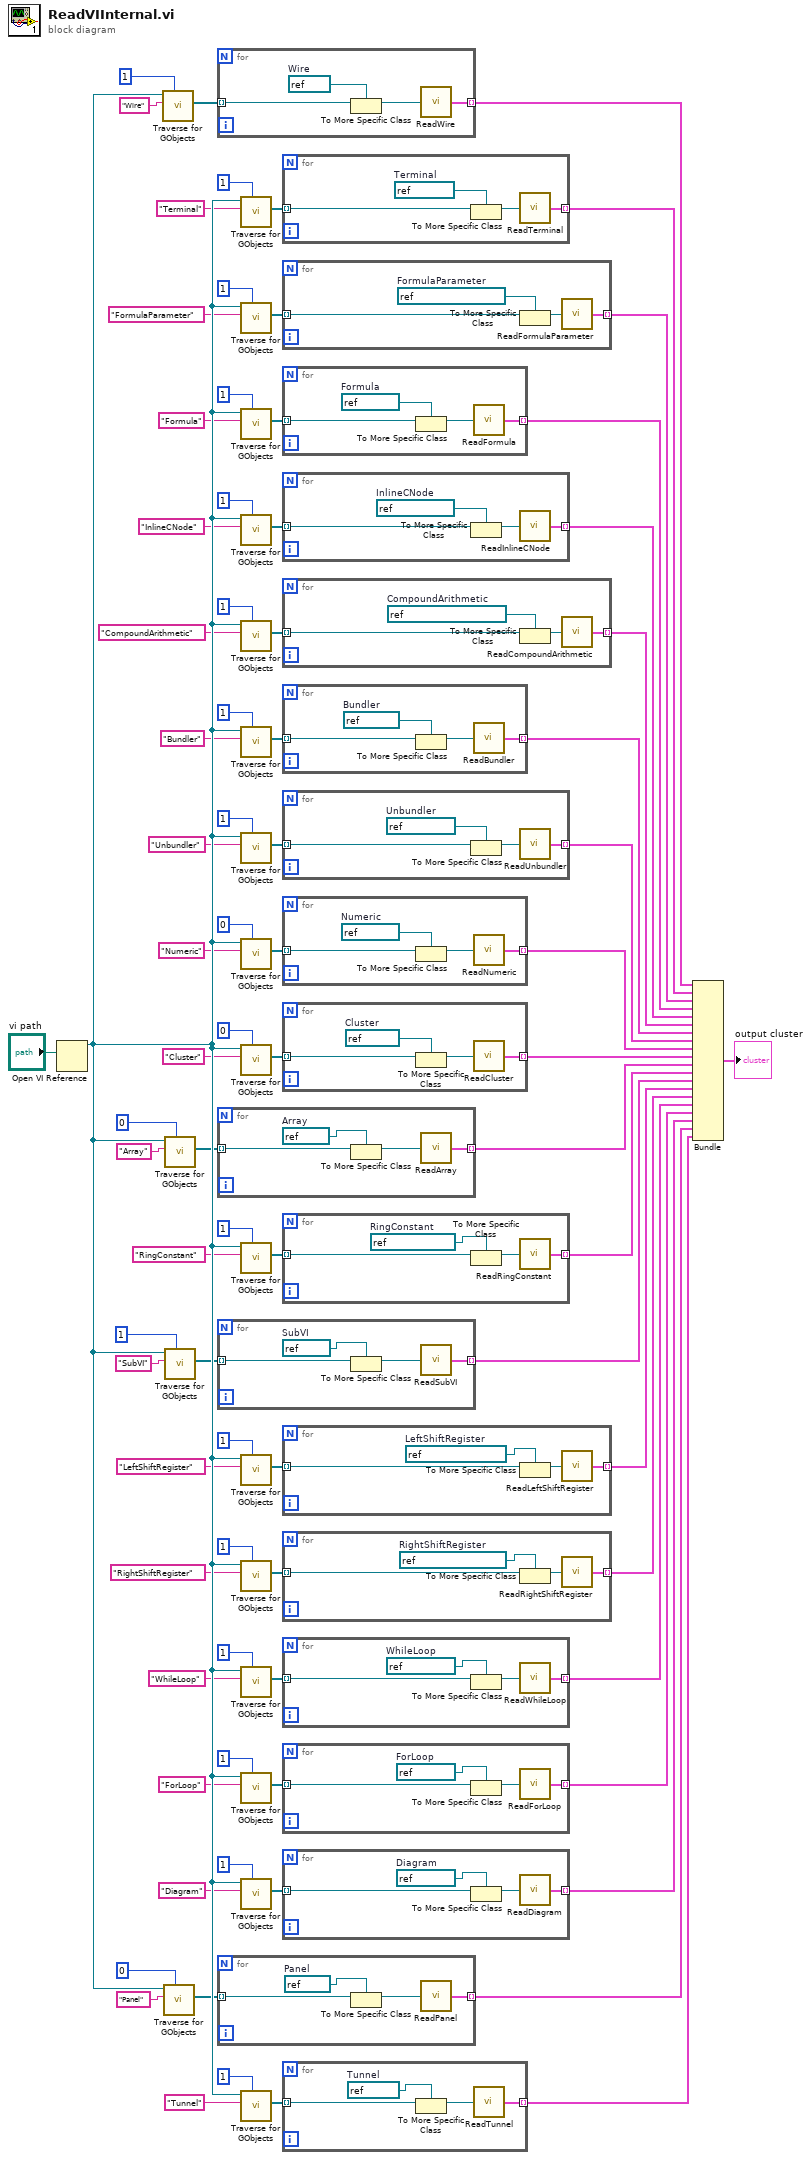
[diagram p0: block diagram]
diagram:
  n1 = Open VI Reference(vi path="vi path") -> (vi reference=w83:refnum<vi>)  [unwired: 5 in, 1 out]
  n2 = call <vilib>:"Traverse for GObjects.vi"("Traverse Target"=1, "Class Name"="Wire", "VI Refnum"=w83) -> ("References"=w81:refnum<vi>[])  [unwired: 5 in, 3 out]
  n3 = call <vilib>:"Traverse for GObjects.vi"("Traverse Target"=0, "Class Name"="Panel", "VI Refnum"=w83) -> ("References"=w9:refnum<vi>[])  [unwired: 5 in, 3 out]
  n4 = call <vilib>:"Traverse for GObjects.vi"("Traverse Target"=0, "Class Name"="Array", "VI Refnum"=w83) -> ("References"=w41:refnum<vi>[])  [unwired: 5 in, 3 out]
  n5 = call <vilib>:"Traverse for GObjects.vi"("Traverse Target"=1, "Class Name"="SubVI", "VI Refnum"=w83) -> ("References"=w33:refnum<vi>[])  [unwired: 5 in, 3 out]
  n6 = for {
    tunnel: w81 -> [w87] mode=indexing
    tunnel: [w85] -> w79 mode=indexing
    w86 = refnum<vi> refnum  # Wire
    n7 = To More Specific Class(target class=w86, reference=w87) -> (specific class reference=w84:refnum<vi>)  [unwired: 1 in, 1 out]
    n8 = call "ReadWire.vi"("reference"=w84) -> ("Wire"=w85:T14)
  }
  n9 = for {
    tunnel: w41 -> [w91] mode=indexing
    tunnel: [w89] -> w39 mode=indexing
    w90 = refnum<vi> refnum  # Array
    n10 = To More Specific Class(target class=w90, reference=w91) -> (specific class reference=w88:refnum<vi>)  [unwired: 1 in, 1 out]
    n11 = call "ReadArray.vi"("reference"=w88) -> ("Array"=w89:T15)
  }
  n12 = for {
    tunnel: w33 -> [w95] mode=indexing
    tunnel: [w93] -> w31 mode=indexing
    w94 = refnum<vi> refnum  # SubVI
    n13 = To More Specific Class(target class=w94, reference=w95) -> (specific class reference=w92:refnum<vi>)  [unwired: 1 in, 1 out]
    n14 = call "ReadSubVI.vi"("reference"=w92) -> ("SubVI"=w93:T16)
  }
  n15 = for {
    tunnel: w9 -> [w99] mode=indexing
    tunnel: [w97] -> w7 mode=indexing
    w98 = refnum<vi> refnum  # Panel
    n16 = To More Specific Class(target class=w98, reference=w99) -> (specific class reference=w96:refnum<vi>)  [unwired: 1 in, 1 out]
    n17 = call "ReadPanel.vi"("reference"=w96) -> ("Panel"=w97:T17)
  }
  n18 = call <vilib>:"Traverse for GObjects.vi"("Traverse Target"=1, "Class Name"="Terminal", "VI Refnum"=w83) -> ("References"=w77:refnum<vi>[])  [unwired: 5 in, 3 out]
  n19 = call <vilib>:"Traverse for GObjects.vi"("Traverse Target"=1, "Class Name"="FormulaParameter", "VI Refnum"=w83) -> ("References"=w73:refnum<vi>[])  [unwired: 5 in, 3 out]
  n20 = call <vilib>:"Traverse for GObjects.vi"("Traverse Target"=1, "Class Name"="Formula", "VI Refnum"=w83) -> ("References"=w69:refnum<vi>[])  [unwired: 5 in, 3 out]
  n21 = call <vilib>:"Traverse for GObjects.vi"("Traverse Target"=1, "Class Name"="InlineCNode", "VI Refnum"=w83) -> ("References"=w65:refnum<vi>[])  [unwired: 5 in, 3 out]
  n22 = call <vilib>:"Traverse for GObjects.vi"("Traverse Target"=1, "Class Name"="CompoundArithmetic", "VI Refnum"=w83) -> ("References"=w61:refnum<vi>[])  [unwired: 5 in, 3 out]
  n23 = call <vilib>:"Traverse for GObjects.vi"("Traverse Target"=1, "Class Name"="Bundler", "VI Refnum"=w83) -> ("References"=w57:refnum<vi>[])  [unwired: 5 in, 3 out]
  n24 = call <vilib>:"Traverse for GObjects.vi"("Traverse Target"=1, "Class Name"="Unbundler", "VI Refnum"=w83) -> ("References"=w54:refnum<vi>[])  [unwired: 5 in, 3 out]
  n25 = call <vilib>:"Traverse for GObjects.vi"("Traverse Target"=0, "Class Name"="Numeric", "VI Refnum"=w83) -> ("References"=w49:refnum<vi>[])  [unwired: 5 in, 3 out]
  n26 = call <vilib>:"Traverse for GObjects.vi"("Traverse Target"=0, "Class Name"="Cluster", "VI Refnum"=w83) -> ("References"=w45:refnum<vi>[])  [unwired: 5 in, 3 out]
  n27 = call <vilib>:"Traverse for GObjects.vi"("Traverse Target"=1, "Class Name"="RingConstant", "VI Refnum"=w83) -> ("References"=w37:refnum<vi>[])  [unwired: 5 in, 3 out]
  n28 = call <vilib>:"Traverse for GObjects.vi"("Traverse Target"=1, "Class Name"="LeftShiftRegister", "VI Refnum"=w83) -> ("References"=w29:refnum<vi>[])  [unwired: 5 in, 3 out]
  n29 = call <vilib>:"Traverse for GObjects.vi"("Traverse Target"=1, "Class Name"="RightShiftRegister", "VI Refnum"=w83) -> ("References"=w25:refnum<vi>[])  [unwired: 5 in, 3 out]
  n30 = call <vilib>:"Traverse for GObjects.vi"("Traverse Target"=1, "Class Name"="WhileLoop", "VI Refnum"=w83) -> ("References"=w21:refnum<vi>[])  [unwired: 5 in, 3 out]
  n31 = call <vilib>:"Traverse for GObjects.vi"("Traverse Target"=1, "Class Name"="ForLoop", "VI Refnum"=w83) -> ("References"=w17:refnum<vi>[])  [unwired: 5 in, 3 out]
  n32 = call <vilib>:"Traverse for GObjects.vi"("Traverse Target"=1, "Class Name"="Diagram", "VI Refnum"=w83) -> ("References"=w13:refnum<vi>[])  [unwired: 5 in, 3 out]
  n33 = call <vilib>:"Traverse for GObjects.vi"("Traverse Target"=1, "Class Name"="Tunnel", "VI Refnum"=w83) -> ("References"=w5:refnum<vi>[])  [unwired: 5 in, 3 out]
  n34 = for {
    tunnel: w77 -> [w103] mode=indexing
    tunnel: [w101] -> w75 mode=indexing
    w102 = refnum<vi> refnum  # Terminal
    n35 = To More Specific Class(target class=w102, reference=w103) -> (specific class reference=w100:refnum<vi>)  [unwired: 1 in, 1 out]
    n36 = call "ReadTerminal.vi"("reference"=w100) -> ("Terminal"=w101:T18)
  }
  n37 = for {
    tunnel: w73 -> [w107] mode=indexing
    tunnel: [w105] -> w71 mode=indexing
    w106 = refnum<vi> refnum  # FormulaParameter
    n38 = To More Specific Class(target class=w106, reference=w107) -> (specific class reference=w104:refnum<vi>)  [unwired: 1 in, 1 out]
    n39 = call "ReadFormulaParameter.vi"("reference"=w104) -> ("FormulaParameter"=w105:T19)
  }
  n40 = for {
    tunnel: w69 -> [w111] mode=indexing
    tunnel: [w109] -> w67 mode=indexing
    w110 = refnum<vi> refnum  # Formula
    n41 = To More Specific Class(target class=w110, reference=w111) -> (specific class reference=w108:refnum<vi>)  [unwired: 1 in, 1 out]
    n42 = call "ReadFormula.vi"("reference"=w108) -> ("Formula"=w109:T20)
  }
  n43 = for {
    tunnel: w65 -> [w115] mode=indexing
    tunnel: [w113] -> w63 mode=indexing
    w114 = refnum<vi> refnum  # InlineCNode
    n44 = To More Specific Class(target class=w114, reference=w115) -> (specific class reference=w112:refnum<vi>)  [unwired: 1 in, 1 out]
    n45 = call "ReadInlineCNode.vi"("reference"=w112) -> ("InlineCNode"=w113:T20)
  }
  n46 = for {
    tunnel: w61 -> [w119] mode=indexing
    tunnel: [w117] -> w59 mode=indexing
    w118 = refnum<vi> refnum  # CompoundArithmetic
    n47 = To More Specific Class(target class=w118, reference=w119) -> (specific class reference=w116:refnum<vi>)  [unwired: 1 in, 1 out]
    n48 = call "ReadCompoundArithmetic.vi"("reference"=w116) -> ("CompoundArithmetic"=w117:T21)
  }
  n49 = for {
    tunnel: w57 -> [w123] mode=indexing
    tunnel: [w121] -> w55 mode=indexing
    w122 = refnum<vi> refnum  # Bundler
    n50 = To More Specific Class(target class=w122, reference=w123) -> (specific class reference=w120:refnum<vi>)  [unwired: 1 in, 1 out]
    n51 = call "ReadBundler.vi"("reference"=w120) -> ("Bundler"=w121:T22)
  }
  n52 = for {
    tunnel: w54 -> [w127] mode=indexing
    tunnel: [w125] -> w51 mode=indexing
    w126 = refnum<vi> refnum  # Unbundler
    n53 = To More Specific Class(target class=w126, reference=w127) -> (specific class reference=w124:refnum<vi>)  [unwired: 1 in, 1 out]
    n54 = call "ReadUnbundler.vi"("reference"=w124) -> ("Unbundler"=w125:T23)
  }
  n55 = for {
    tunnel: w49 -> [w131] mode=indexing
    tunnel: [w129] -> w47 mode=indexing
    w130 = refnum<vi> refnum  # Numeric
    n56 = To More Specific Class(target class=w130, reference=w131) -> (specific class reference=w128:refnum<vi>)  [unwired: 1 in, 1 out]
    n57 = call "ReadNumeric.vi"("reference"=w128) -> ("Numeric"=w129:T24)
  }
  n58 = for {
    tunnel: w45 -> [w135] mode=indexing
    tunnel: [w133] -> w43 mode=indexing
    w134 = refnum<vi> refnum  # Cluster
    n59 = To More Specific Class(target class=w134, reference=w135) -> (specific class reference=w132:refnum<vi>)  [unwired: 1 in, 1 out]
    n60 = call "ReadCluster.vi"("reference"=w132) -> ("Cluster"=w133:T25)
  }
  n61 = for {
    tunnel: w37 -> [w139] mode=indexing
    tunnel: [w137] -> w35 mode=indexing
    w138 = refnum<vi> refnum  # RingConstant
    n62 = To More Specific Class(target class=w138, reference=w139) -> (specific class reference=w136:refnum<vi>)  [unwired: 1 in, 1 out]
    n63 = call "ReadRingConstant.vi"("reference"=w136) -> ("RingConstant"=w137:T26)
  }
  n64 = for {
    tunnel: w29 -> [w143] mode=indexing
    tunnel: [w141] -> w27 mode=indexing
    w142 = refnum<vi> refnum  # LeftShiftRegister
    n65 = To More Specific Class(target class=w142, reference=w143) -> (specific class reference=w140:refnum<vi>)  [unwired: 1 in, 1 out]
    n66 = call "ReadLeftShiftRegister.vi"("reference"=w140) -> ("LeftShiftRegister"=w141:T27)
  }
  n67 = for {
    tunnel: w25 -> [w147] mode=indexing
    tunnel: [w145] -> w23 mode=indexing
    w146 = refnum<vi> refnum  # RightShiftRegister
    n68 = To More Specific Class(target class=w146, reference=w147) -> (specific class reference=w144:refnum<vi>)  [unwired: 1 in, 1 out]
    n69 = call "ReadRightShiftRegister.vi"("reference"=w144) -> ("RightShiftRegister"=w145:T28)
  }
  n70 = for {
    tunnel: w21 -> [w151] mode=indexing
    tunnel: [w149] -> w19 mode=indexing
    w150 = refnum<vi> refnum  # WhileLoop
    n71 = To More Specific Class(target class=w150, reference=w151) -> (specific class reference=w148:refnum<vi>)  [unwired: 1 in, 1 out]
    n72 = call "ReadWhileLoop.vi"("reference"=w148) -> ("WhileLoop"=w149:T29)
  }
  n73 = for {
    tunnel: w17 -> [w155] mode=indexing
    tunnel: [w153] -> w15 mode=indexing
    w154 = refnum<vi> refnum  # ForLoop
    n74 = To More Specific Class(target class=w154, reference=w155) -> (specific class reference=w152:refnum<vi>)  [unwired: 1 in, 1 out]
    n75 = call "ReadForLoop.vi"("reference"=w152) -> ("ForLoop"=w153:T30)
  }
  n76 = for {
    tunnel: w13 -> [w159] mode=indexing
    tunnel: [w157] -> w11 mode=indexing
    w158 = refnum<vi> refnum  # Diagram
    n77 = To More Specific Class(target class=w158, reference=w159) -> (specific class reference=w156:refnum<vi>)  [unwired: 1 in, 1 out]
    n78 = call "ReadDiagram.vi"("reference"=w156) -> ("Diagram"=w157:T31)
  }
  n79 = for {
    tunnel: w5 -> [w163] mode=indexing
    tunnel: [w161] -> w3 mode=indexing
    w162 = refnum<vi> refnum  # Tunnel
    n80 = To More Specific Class(target class=w162, reference=w163) -> (specific class reference=w160:refnum<vi>)  [unwired: 1 in, 1 out]
    n81 = call "ReadTunnel.vi"("reference"=w160) -> ("Tunnel"=w161:T32)
  }
  n82 = Bundle(w79, w75, w71, w67, w63, w59, w55, w51, w47, w43, w39, w35, w31, w27, w23, w19, w15, w11, w7, w3) -> (→"output cluster":T33)  [unwired: 1 in]
